vi "HideFrontPanel.vi"(8 "error in (no error)":errorcluster, 11 "Gui in":refnum<class "Gui.lvclass">) -> (0 "error out":errorcluster, 3 "Gui out":refnum<class "Gui.lvclass">)   [LabVIEW 2022 SP3, in "Gui.lvlib" / "Gui.lvclass"]
uses:
  Gui.lvclass
  Gui.lvclass/Gui.ctl
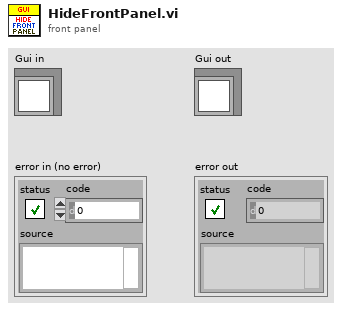
[diagram p1: front panel]
types:
  T1 = enum32{"Invalid", "Standard", "Closed", "Hidden", "Minimized", "Maximized"}
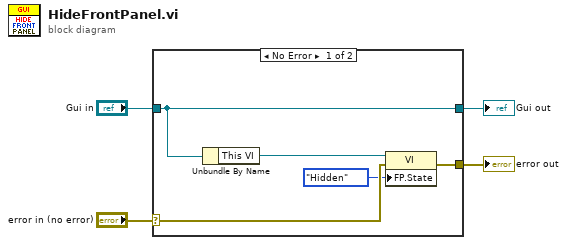
[diagram p0: block diagram]
diagram:
  n1 = case shown="No Error" "error in (no error)" {
    selector: "error in (no error)" -> [w7 w11]
    tunnel: [w6 w11] -> w3
    tunnel: [w9 w10] -> w1
    tunnel: "Gui in" -> [w9 w10]
    frame No Error {
      n2 = Unbundle By Name(w9) -> ("This VI"=w8:refnum<vi>)
      n3 = property class="VI"(reference=w8, error in=w7, "FP.State"=T1."Hidden" ("Front Panel Window:State")) -> (error out=w6:errorcluster)  [unwired: 1 out]
    }
    frame Error {
    }
  }
  "error out" <- w3
  "Gui out" <- w1
